vi "Adept - Flash FPGA Bitfile.vi"() -> ()   [LabVIEW 2011]
uses:
  vi.lib/LabVIEW Hacker/Adept/Private/Type Defs/Adept Device Ctl.xctl
  vi.lib/LabVIEW Hacker/Adept/LVH-Adept.lvlib
panel:
  out "Status":string
  in  "Bit File Path":path
  in  "Adept Device":u16(xcontrol)
  # "Configuration"
  # "Status"
  # "Load Bitfile\n\nThis example demonstrates how to flash bitfile to a Digilent FPGA board.\n\nInstructions\n1. Select the Adept Device.\n2. Click the Bitfile Path browse button.\n4. Click the Run Arrow.\n5. Notice the Status changes to indicate when the operation is complete."
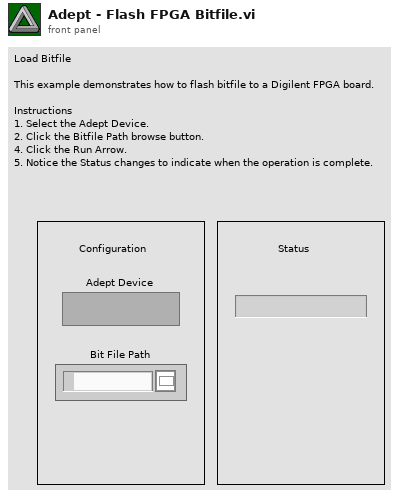
[diagram p1: front panel]
types:
  T1 = typedef "LVH-Adept.lvlib/Device Config.ctl" = cluster{"Num Devices":i32, "Device Names":string[], "Device Index":u16, "Device Handle":u32, "Status":T2}
  T2 = typedef "LVH-Adept.lvlib/Status.ctl" = cluster{"DEPP":bool, "DSTM":bool, "DJTG":bool}
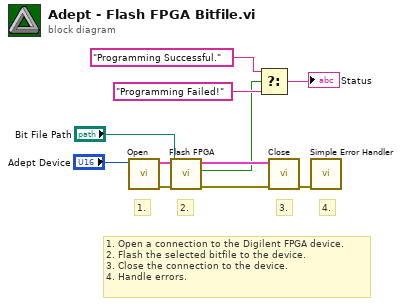
[diagram p0: block diagram]
diagram:
  # "1. Open a connection to the Digilent FPGA device.\n2. Flash the selected bitfile to the device.\n3. Close the connection to the device.\n4. Handle errors."
  # "4."
  # "3."
  # "2."
  # "1."
  n1 = call "Open.vi"("Adept Device"="Adept Device") -> ("Error Out"=w10:errorcluster, "Adept Config"=w11:T1)  [unwired: 9 in]
  n2 = call "Flash FPGA.vi"("Error In"=w10, "Bit File Path"="Bit File Path", "Adept Config"=w11) -> ("Error Out"=w9:errorcluster, "Success?"=w4:bool, "Adept Config"=w8:T1)  [unwired: 6 in]
  n3 = Select(t="Programming Successful.", s=w4, f="Programming Failed!") -> (s? t:f=→"Status":string)
  n4 = call "Close.vi"("Error In"=w9, "Adept Config"=w8) -> ("Error Out"=w7:errorcluster)  [unwired: 9 in]
  n5 = call <vilib>:"Simple Error Handler.vi"("error in (no error)"=w7) -> ()  [unwired: 4 in, 5 out]
